vi "ParseData.vi"(11 "DATA":string(combo)="ATDATA") -> (3 "data":dbl[](array[numeric]))   [LabVIEW 2011]
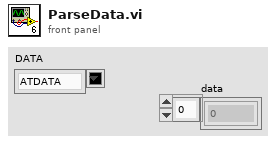
[diagram p1: front panel]
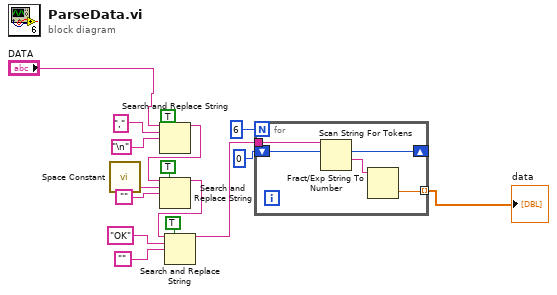
[diagram p0: block diagram]
diagram:
  n1 = call <vilib>:"Space Constant.vi"() -> ("String"=w7:string)
  n2 = Search and Replace String(replace all?=TRUE ("replace all? (F)"), input string="DATA", search string=",", replace string="\n") -> (result string=w8:string)  [unwired: 4 in, 3 out]
  n3 = Search and Replace String(replace all?=TRUE ("replace all? (F)"), input string=w8, search string=w7, replace string="") -> (result string=w11:string)  [unwired: 4 in, 3 out]
  n4 = Search and Replace String(replace all?=TRUE ("replace all? (F)"), input string=w11, search string="OK" ("substring (\"\")"), replace string="") -> (result string=w3:string)  [unwired: 4 in, 3 out]
  n5 = for {
    N: 6 -> [_]
    shift-right: [w20] -> _
    shift-left: 0 ("offset of match") -> [w21]
    tunnel: w3 -> [w19]
    tunnel: [w18] -> w1 mode=indexing
    n6 = Scan String For Tokens(8:w21, 9:w19) -> (1:w17:string, 2:w20:i32)  [unwired: 4 in, 2 out]
    n7 = Fract/Exp String To Number(string=w17) -> (number=w18:dbl)  [unwired: 3 in, 1 out]
  }
  "data" <- w1
